vi "format_NM_pt_history.vi"(8 "path-in":path=path "C:/Users/hpDIRC/Desktop/Tyler/t3.csv", 9 "trial #":i32, 11 "data in":dbl[][](array[numeric])) -> ()   [LabVIEW 2024]
uses:
  2cff1179-351a-4d85-a51f-5a8fa7e98cb1.vi
panel:
  in  "GrAsc in":dbl[][](array[numeric])
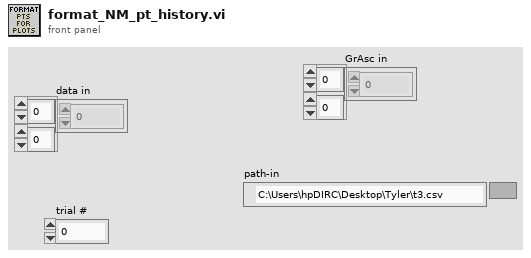
[diagram p1: front panel]
types:
  T1 = enum16{"open", "replace", "create", "open or create", "replace or create", "replace or create with confirmation"}
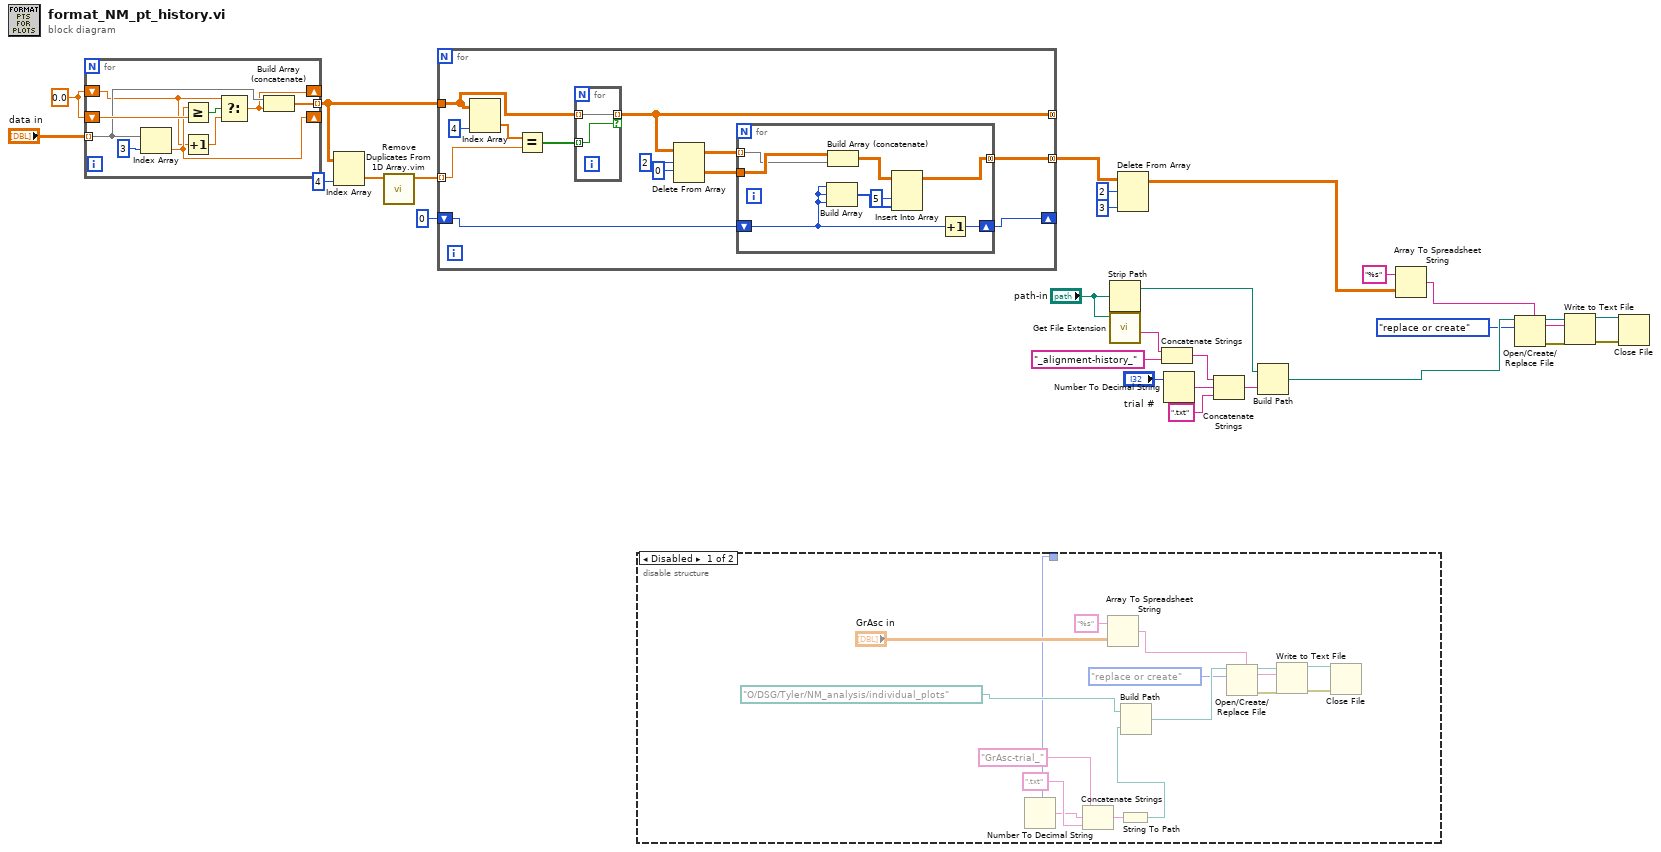
[diagram p0: block diagram]
diagram:
  w16 = 0.0
  n1 = for {
    tunnel: "data in" -> [w35] mode=indexing
    shift-right: [w34] -> _
    shift-left: w16 -> [w36]
    tunnel: [w33] -> w20 mode=indexing
    shift-right: [w29] -> _
    shift-left: w16 -> [w31]
    n2 = Index Array(array=w35, index=3) -> (element=w34:dbl)
    n3 = Greater Or Equal?(x=w34, y=w36) -> (x >= y?=w32:bool)
    n4 = Increment(x=w31) -> (x+1=w30:dbl)
    n5 = Select(t=w31, s=w32, f=w30) -> (s? t:f=w29:dbl)
    n6 = Build Array (concatenate)(w35, w29) -> (w33:dbl[])
  }
  n7 = Index Array(array=w20, index (col)=4 ("disabled index (col)")) -> (element=w18:dbl[])  [unwired: 1 in]
  n8 = call "Remove Duplicates From 1D Array.vim"("array"=w18) -> ("array with duplicates removed"=w19:dbl[])  [unwired: 10 in]
  n9 = for {
    tunnel: w19 -> [w48] mode=indexing
    tunnel: w20 -> [w46]
    tunnel: [w38] -> _ mode=concatenating
    tunnel: [w41] -> w22 mode=concatenating
    shift-right: [w39] -> _
    shift-left: 0 -> [w40]
    n10 = Index Array(array=w46, index (col)=4 ("disabled index (col)")) -> (element=w49:dbl[])  [unwired: 1 in]
    n11 = Equal?(x=w49, y=w48) -> (x = y?=w47:bool[])
    n12 = for {
      tunnel: w47 -> [w59] mode=indexing
      tunnel: w46 -> [w60] mode=indexing
      tunnel: [w60] -> w38 mode=indexing if=w59
    }
    n13 = Delete From Array(array=w38, length=2, index (row)=0) -> (deleted portion=w42:dbl[][], array with subset deleted=w43:dbl[][])  [unwired: 1 in]
    n14 = for {
      tunnel: w43 -> [w57] mode=indexing
      tunnel: w42 -> [w58]
      tunnel: [w55] -> w41 mode=concatenating
      shift-right: [w51] -> w39
      shift-left: w40 -> [w52]
      n15 = Build Array(w52, w52, w52) -> (w54:i32[])
      n16 = Build Array (concatenate)(w58, w57) -> (w56:dbl[][])
      n17 = Insert Into Array(array=w56, index (col)=5 ("disabled index (col)"), new element=w54) -> (w55:dbl[][])  [unwired: 1 in]
      n18 = Increment(x=w52) -> (x+1=w51:i32)
    }
  }
  n19 = disable-structure shown="Disabled" {
    disable-tunnel: _ -> [w61 _]
    frame Disabled {
      n20 = Number To Decimal String(number=w61) -> (decimal integer string=w63:string)  [unwired: 1 in]
      n21 = Concatenate Strings("GrAsc-trial_" ("string"), w63, ".txt" ("string")) -> (w71:string)
      n22 = Array To Spreadsheet String(array="GrAsc in", 3:"%s" ("format string")) -> (spreadsheet string=w74:string)  [unwired: 1 in]
      n23 = String To Path(string=w71) -> (path=w72:path)
      n24 = Build Path(base path=path "O:/DSG/Tyler/NM_analysis/individual_plots", name or relative path=w72) -> (appended path=w73:path)
      n25 = Open/Create/Replace File(file path (use dialog)=w73, operation (0:open)=T1."replace or create") -> (refnum out=w67:refnum<file>, error out=w66:errorcluster)  [unwired: 4 in, 1 out]
      n26 = Write to Text File(file (use dialog)=w67, text=w74, error in=w66) -> (refnum out=w68:refnum<file>, error out=w69:errorcluster)  [unwired: 1 in, 1 out]
      n27 = Close File(refnum=w68, error in=w69) -> ()  [unwired: 2 out]
    }
    frame Enabled {
    }
  }
  n28 = Strip Path(path="path-in") -> (stripped path=w10:path)  [unwired: 1 out]
  n29 = call <vilib>:"Get File Extension.vi"("file"="path-in") -> ("filename without extension"=w13:string)  [unwired: 6 in, 4 out]
  n30 = Delete From Array(array=w22, length=2, index (col)=3 ("disabled index (col)")) -> (array with subset deleted=w27:dbl[][])  [unwired: 1 in, 1 out]
  n31 = Concatenate Strings(w13, "_alignment-history_" ("string")) -> (w11:string)
  n32 = Number To Decimal String(number="trial #") -> (decimal integer string=w25:string)  [unwired: 1 in]
  n33 = Concatenate Strings(w11, w25, ".txt" ("string")) -> (w9:string)
  n34 = Build Path(base path=w10, name or relative path=w9) -> (appended path=w8:path)
  n35 = Array To Spreadsheet String(array=w27, 3:"%s" ("format string")) -> (spreadsheet string=w7:string)  [unwired: 1 in]
  n36 = Open/Create/Replace File(file path (use dialog)=w8, operation (0:open)=T1."replace or create") -> (refnum out=w3:refnum<file>, error out=w2:errorcluster)  [unwired: 4 in, 1 out]
  n37 = Write to Text File(file (use dialog)=w3, text=w7, error in=w2) -> (refnum out=w4:refnum<file>, error out=w5:errorcluster)  [unwired: 1 in, 1 out]
  n38 = Close File(refnum=w4, error in=w5) -> ()  [unwired: 2 out]
